vi "Get Hash Info.vi"(8 "error in (no error)":errorcluster, 11 "SHA-1 in":refnum<class "SHA-1.lvclass">) -> (0 "error out":errorcluster, 1 "Output Length (Bytes)":i32, 2 "Blocksize (Bytes)":i32, 3 "SHA-1 out":refnum<class "SHA-1.lvclass">)   [LabVIEW 2020, in "Crypto.lvlib" / "SHA-1.lvclass"]
uses:
  SHA-1.lvclass
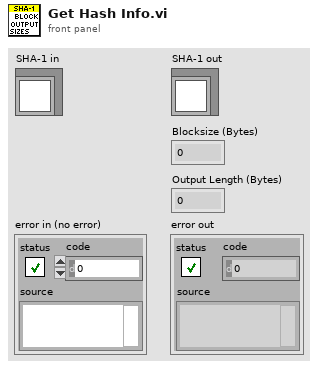
[diagram p1: front panel]
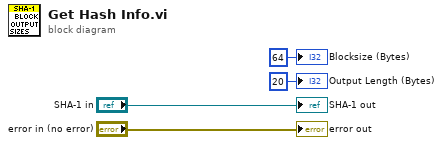
[diagram p0: block diagram]
diagram:
  "error out" <- "error in (no error)"
  "SHA-1 out" <- "SHA-1 in"
  "Blocksize (Bytes)" <- 64 ("Blocksize (Bytes)")
  "Output Length (Bytes)" <- 20 ("Output Length (Bytes)")
